vi "Teleop.vi"(10 "Match Info":T1={"Autonomous Elapsed Seconds"=0.0, "TeleOp Elapsed Seconds"=0.0, "Disabled Elapsed Seconds"=0.0, "Visited Autonomous"=FALSE, "Visited TeleOp"=FALSE, "Visited Disabled"=FALSE, "Autonomous Settings"={"Autonomous Style"=enum."Independent", "VI Refnum"=refnum}}, 11 "Call Context":T2) -> ()   [LabVIEW 2011]
doc: "This VI is called for each TeleOp packet received from the DS where the robot is not disabled. It is often used to read from the joysticks and update I/O or to update setpoints for timed control loops. It should complete and return within 20 milliseconds or it may miss DS packets."
uses:
  <vilib>/Rock Robotics/WPI/DriverStation/WPI_DriverStationDerivedRobotMode.ctl
  <vilib>/Rock Robotics/WPI/DriverStation/WPI_DriverStationMatch Info.ctl
  Robot Global Data.vi
panel:
  in  "Turret":dbl(knob)=0.008480890251286732 scale=-1.0..1.0
  out "Turret Output":dbl
  in  "Conveyor":dbl(knob) scale=-0.1..1.0
  out "Conveyor Output":dbl
  in  "Harvester":dbl(knob) scale=-1.0..1.0
  out "Harvester Output":dbl
  out "Shooter Output":dbl
  in  "Shooter":dbl(knob) scale=0.0..1.0
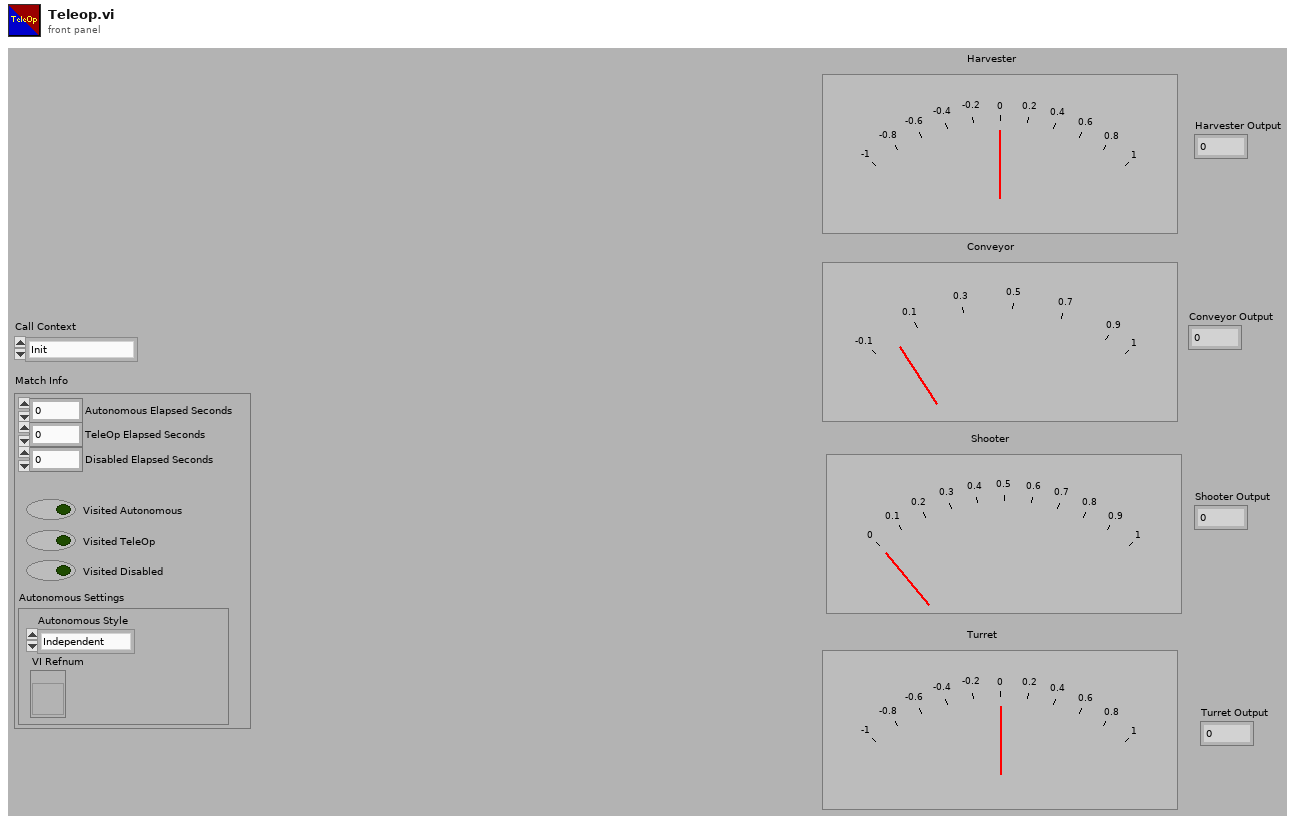
[diagram p1: front panel]
types:
  T1 = typedef "WPI_DriverStationMatch Info.ctl" = cluster{"Autonomous Elapsed Seconds":dbl, "TeleOp Elapsed Seconds":dbl, "Disabled Elapsed Seconds":dbl, "Visited Autonomous":bool, "Visited TeleOp":bool, "Visited Disabled":bool, "Autonomous Settings":cluster{"Autonomous Style":enum16{"Iterative", "Independent"}, "VI Refnum":refnum<vi>}}
  T2 = typedef "WPI_DriverStationDerivedRobotMode.ctl" = enum16{"Init", "Execute", "Stop"}
  T3 = typedef "WPI_JoystickDevRef.ctl" = cluster{"Device":T4}
  T4 = typedef "WPI_JoystickDeviceEnum.ctl" = enum16{"USB 1", "USB 2", "USB 3", "USB 4", "Kinect 1", "Kinect 2"}
  T5 = typedef "WPI_JoystickButtonState.ctl" = cluster{"Button 1":bool, "Button 2":bool, "Button 3":bool, "Button 4":bool, "Button 5":bool, "Button 6":bool, "Button 7":bool, "Button 8":bool, "Button 9":bool, "Button 10":bool, "Button 11":bool, "Button 12":bool}
  T6 = typedef "WPI_DigitalInputDevRef.ctl" = cluster{"DevStatus":errorcluster, "DIO Channel":T7, "Digital Module":T8}
  T7 = typedef "FPGA_DIOChannel.ctl" = enum8{"DIO 1", "DIO 2", "DIO 3", "DIO 4", "DIO 5", "DIO 6", "DIO 7", "DIO 8", "DIO 9", "DIO 10", "DIO 11", "DIO 12", "DIO 13", "DIO 14", "Invalid"}
  T8 = typedef "FPGA_TypedefDigitalModule.ctl" = enum16{"Digital Module 1", "Digital Module 2"}
  T9 = cluster{"Driver Station Digital Output (1-8)[0]":bool, "Driver Station Digital Output (1-8)[1]":bool, "Driver Station Digital Output (1-8)[2]":bool, "Driver Station Digital Output (1-8)[3]":bool, "Driver Station Digital Output (1-8)[4]":bool, "Driver Station Digital Output (1-8)[5]":bool, "Driver Station Digital Output (1-8)[6]":bool, "Driver Station Digital Output (1-8)[7]":bool, "Driver Station Digital Output (1-8)[8]":bool}
  T10 = cluster{"axis 1 (x)":dbl, "axis 2 (y)":dbl, "axis 3 (throttle)":dbl, "axis 4":dbl, "axis 5":dbl, "axis 6":dbl}
  T11 = typedef "WPI_ServoDeviceRef.ctl" = cluster{"DeviceStatus":errorcluster, "Digital Module":T8, "PWM Channel":T12, "DeadBand":T13}
  T12 = typedef "FPGA_DIOPWMChannel.ctl" = enum8{"PWM 1", "PWM 2", "PWM 3", "PWM 4", "PWM 5", "PWM 6", "PWM 7", "PWM 8", "PWM 9", "PWM 10", "Invalid"}
  T13 = typedef "WPI_PWMDeadband.ctl" = cluster{"Name":string, "maxPositivePwm":i32, "minPositivePwm":i32, "centerPwm":i32, "maxNegativePwm":i32, "minNegativePwm":i32, "angularRange":u16}
  T14 = typedef "WPI_MotorControlDeviceRef.ctl" = cluster{"DeviceStatus":errorcluster, "Type":enum16{"PWM", "CAN"}, "PWM":cluster{"Digital Module":T8, "PWM Channel":T12, "DeadBand":T13}, "CAN":cluster{"Device Number":u8, "Control Mode":T15, "Semaphore":T16, "Max Vout":dbl}, "Invert":bool, "TransformRef":T17, "InvTransformRef":T17}
  T15 = typedef "WPI_CANJaguar_ControlMode.ctl" = enum8{"Percent VBus", "Current", "Speed", "Position", "Voltage"}
  T16 = typedef "Semaphore RefNum" = refnum<k1>
  T17 = typedef "WPI_PWMTransform_ConPane.ctl" = refnum<vi>
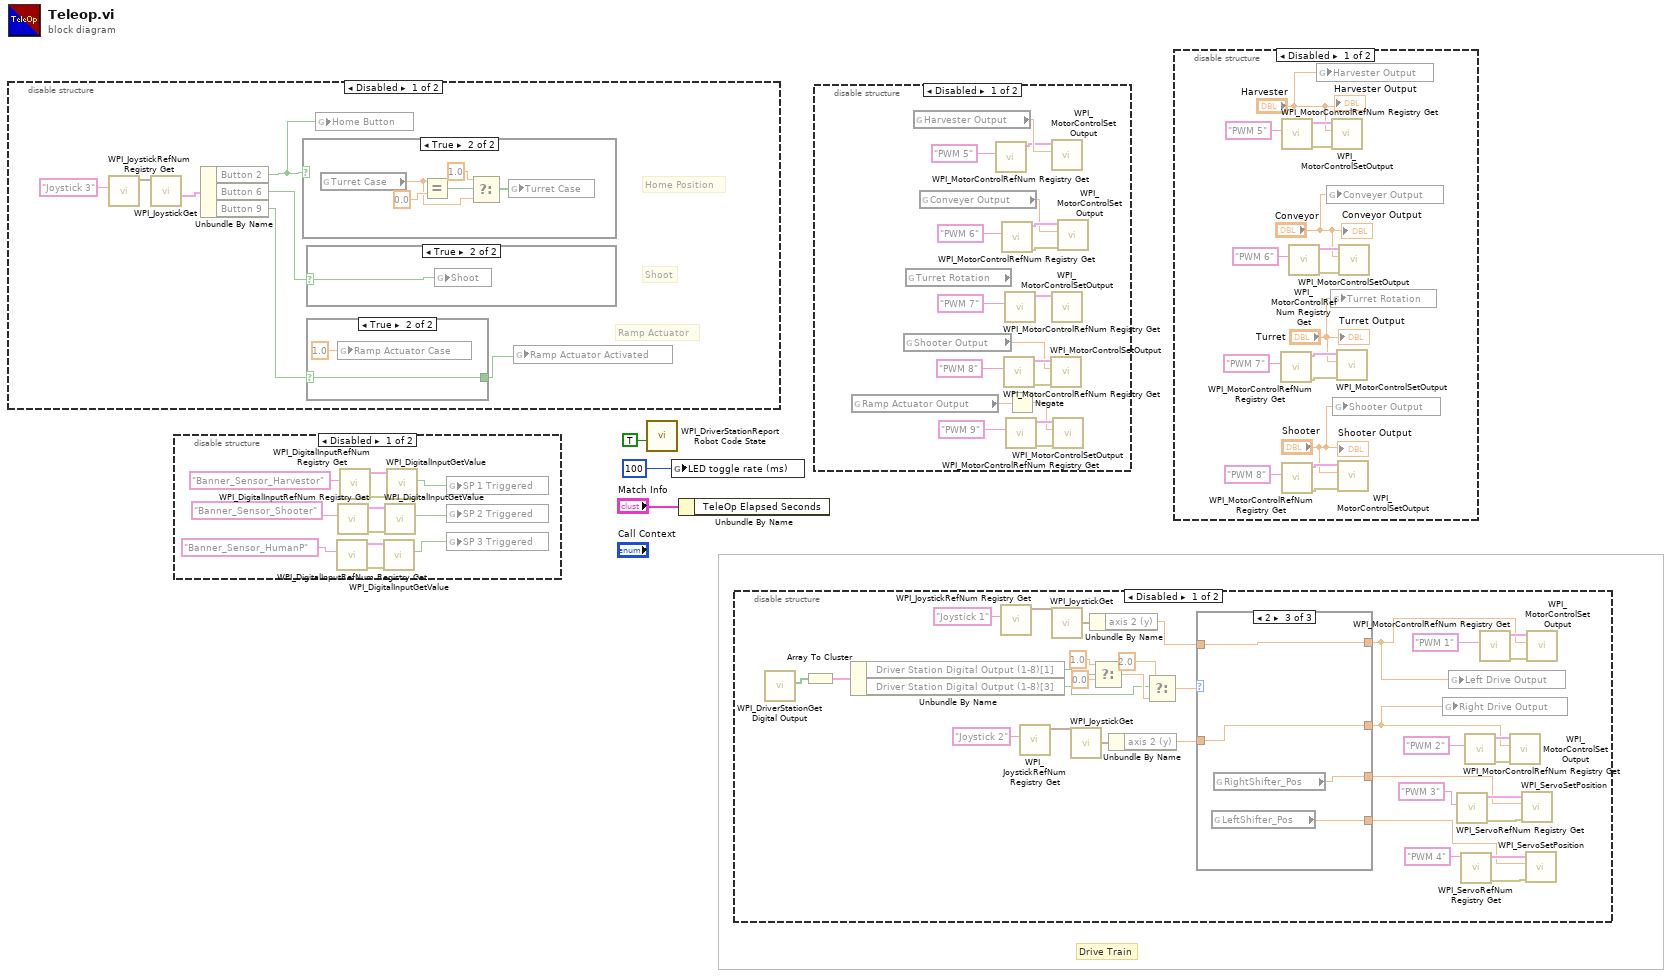
[diagram p0: block diagram]
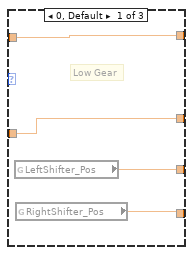
[diagram p3: hidden frame]
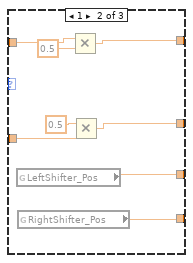
[diagram p4: hidden frame]
diagram:
  # "Drive Train"
  n1 = disable-structure shown="Disabled" {
    frame Disabled {
      # "Ramp Actuator"
      # "Shoot"
      # "Home Position"
      n2 = call <vilib>:"WPI_JoystickRefNum Registry Get.vi"("refnum name"="Joystick 3") -> ("JoystickDevRef"=w7:T3)  [unwired: 9 in, 1 out]
      n3 = call <vilib>:"WPI_JoystickGet.vi"("JoystickDevRef"=w7) -> ("Buttons"=w8:T5)  [unwired: 4 in, 2 out]
      n4 = Unbundle By Name(w8) -> ("Button 2"=w6:bool, "Button 6"=w5:bool, "Button 9"=w4:bool)
      n5 = case shown="True" w6 {
        frame False {
        }
        frame True {
          n6 = global read "Robot Global Data.vi" "Turret Case"() -> (w12:dbl)
          n7 = Equal?(x=w12, y=0.0) -> (x = y?=w14:bool)
          n8 = Select(t=1.0, s=w14, f=w12) -> (s? t:f=w11:dbl)
          n9 = global write "Robot Global Data.vi" "Turret Case"(w11) -> ()
        }
      }
      n10 = case shown="True" w5 {
        selector: w5 -> [_ w16]
        frame False {
        }
        frame True {
          n11 = global write "Robot Global Data.vi" "Shoot"(w16) -> ()
        }
      }
      n12 = case shown="True" w4 {
        selector: w4 -> [w17 w19]
        tunnel: [w17 w19] -> w10
        frame False {
        }
        frame True {
          n13 = global write "Robot Global Data.vi" "Ramp Actuator Case"(1.0 ("Ramp Actuator Case")) -> ()
        }
      }
      n14 = global write "Robot Global Data.vi" "Home Button"(w6) -> ()
      n15 = global write "Robot Global Data.vi" "Ramp Actuator Activated"(w10) -> ()
    }
    frame Enabled {
    }
  }
  n16 = disable-structure shown="Disabled" {
    frame Disabled {
      n17 = call <vilib>:"WPI_DigitalInputRefNum Registry Get.vi"("refnum name"="Banner_Sensor_HumanP") -> ("error out"=w26:errorcluster, "DigitalInputDevRef"=w25:T6)  [unwired: 9 in]
      n18 = call <vilib>:"WPI_DigitalInputRefNum Registry Get.vi"("refnum name"="Banner_Sensor_Shooter") -> ("error out"=w27:errorcluster, "DigitalInputDevRef"=w28:T6)  [unwired: 9 in]
      n19 = call <vilib>:"WPI_DigitalInputRefNum Registry Get.vi"("refnum name"="Banner_Sensor_Harvestor") -> ("error out"=w31:errorcluster, "DigitalInputDevRef"=w30:T6)  [unwired: 9 in]
      n20 = call <vilib>:"WPI_DigitalInputGetValue.vi"("error in (no error)"=w26, "DigitalInputDevRef"=w25) -> ("Value"=w23:bool)  [unwired: 7 in, 2 out]
      n21 = call <vilib>:"WPI_DigitalInputGetValue.vi"("error in (no error)"=w27, "DigitalInputDevRef"=w28) -> ("Value"=w24:bool)  [unwired: 7 in, 2 out]
      n22 = call <vilib>:"WPI_DigitalInputGetValue.vi"("error in (no error)"=w31, "DigitalInputDevRef"=w30) -> ("Value"=w29:bool)  [unwired: 7 in, 2 out]
      n23 = global write "Robot Global Data.vi" "SP 1 Triggered"(w29) -> ()
      n24 = global write "Robot Global Data.vi" "SP 2 Triggered"(w24) -> ()
      n25 = global write "Robot Global Data.vi" "SP 3 Triggered"(w23) -> ()
    }
    frame Enabled {
    }
  }
  n26 = call <vilib>:"WPI_DriverStationReport Robot Code State.vi"("TeleOp"=TRUE ("Autonomous")) -> ()  [unwired: 10 in, 1 out]
  n27 = global write "Robot Global Data.vi" "LED toggle rate (ms)"(u32 100 ("LED ms toggle rate")) -> ()
  n28 = Unbundle By Name("Match Info") -> ()  [unwired: 1 out]
  n29 = disable-structure shown="Disabled" {
    frame Disabled {
      n30 = call <vilib>:"WPI_DriverStationGet Digital Output.vi"() -> ("Driver Station Digital Output (1-8)"=w64:bool[])  [unwired: 10 in, 1 out]
      n31 = Array To Cluster(array=w64) -> (cluster=w63:T9)
      n32 = Unbundle By Name(w63) -> ("Driver Station Digital Output (1-8)[1]"=w32:bool, "Driver Station Digital Output (1-8)[3]"=w59:bool)
      n33 = call <vilib>:"WPI_JoystickRefNum Registry Get.vi"("refnum name"="Joystick 1") -> ("JoystickDevRef"=w55:T3)  [unwired: 9 in, 1 out]
      n34 = call <vilib>:"WPI_JoystickRefNum Registry Get.vi"("refnum name"="Joystick 2") -> ("JoystickDevRef"=w52:T3)  [unwired: 9 in, 1 out]
      n35 = call <vilib>:"WPI_JoystickGet.vi"("JoystickDevRef"=w55) -> ("Axes"=w54:T10)  [unwired: 4 in, 2 out]
      n36 = call <vilib>:"WPI_JoystickGet.vi"("JoystickDevRef"=w52) -> ("Axes"=w53:T10)  [unwired: 4 in, 2 out]
      n37 = Unbundle By Name(w54) -> ("axis 2 (y)"=w49:dbl)
      n38 = Select(t=1.0, s=w32, f=0.0 ("t")) -> (s? t:f=w60:dbl)
      n39 = Unbundle By Name(w53) -> ("axis 2 (y)"=w50:dbl)
      n40 = Select(t=2.0, s=w59, f=w60) -> (s? t:f=w57:dbl)
      n41 = case shown="2" w57 {
        tunnel: w50 -> [w68 w72 w79]
        tunnel: w49 -> [w67 w75 w80]
        tunnel: [w68 w73 w79] -> w41
        tunnel: [w67 w74 w80] -> w42
        tunnel: [w66 w69 w78] -> w34
        tunnel: [w65 w70 w77] -> w33
        frame 0, Default {
          # "Low Gear"
          n42 = global read "Robot Global Data.vi" "LeftShifter_Pos"() -> (w66:dbl)
          n43 = global read "Robot Global Data.vi" "RightShifter_Pos"() -> (w65:dbl)
        }
        frame 1 {
          n44 = global read "Robot Global Data.vi" "LeftShifter_Pos"() -> (w69:dbl)
          n45 = global read "Robot Global Data.vi" "RightShifter_Pos"() -> (w70:dbl)
          n46 = Multiply(x=w75, y=0.5) -> (x*y=w74:dbl)
          n47 = Multiply(x=0.5 ("y"), y=w72) -> (x*y=w73:dbl)
        }
        frame 2 {
          n48 = global read "Robot Global Data.vi" "LeftShifter_Pos"() -> (w77:dbl)
          n49 = global read "Robot Global Data.vi" "RightShifter_Pos"() -> (w78:dbl)
        }
      }
      n50 = global write "Robot Global Data.vi" "Right Drive Output"(w41) -> ()
      n51 = global write "Robot Global Data.vi" "Left Drive Output"(w42) -> ()
      n52 = call <vilib>:"WPI_ServoRefNum Registry Get.vi"("refnum name"="PWM 3") -> ("error out"=w38:errorcluster, "ServoDeviceRef"=w39:T11)  [unwired: 9 in]
      n53 = call <vilib>:"WPI_ServoRefNum Registry Get.vi"("refnum name"="PWM 4") -> ("error out"=w37:errorcluster, "ServoDeviceRef"=w36:T11)  [unwired: 9 in]
      n54 = call <vilib>:"WPI_MotorControlRefNum Registry Get.vi"("refnum name"="PWM 2") -> ("error out"=w43:errorcluster, "MotorControlDevRef"=w44:T14)  [unwired: 9 in]
      n55 = call <vilib>:"WPI_MotorControlRefNum Registry Get.vi"("refnum name"="PWM 1") -> ("error out"=w45:errorcluster, "MotorControlDevRef"=w46:T14)  [unwired: 9 in]
      n56 = call <vilib>:"WPI_MotorControlSetOutput.vi"("error in (no error)"=w43, "Output"=w41, "MotorControlDevRef"=w44) -> ()  [unwired: 7 in, 2 out]
      n57 = call <vilib>:"WPI_ServoSetPosition.vi"("error in (no error)"=w38, "Position"=w34, "ServoDeviceRef"=w39) -> ()  [unwired: 7 in, 2 out]
      n58 = call <vilib>:"WPI_ServoSetPosition.vi"("error in (no error)"=w37, "Position"=w33, "ServoDeviceRef"=w36) -> ()  [unwired: 7 in, 2 out]
      n59 = call <vilib>:"WPI_MotorControlSetOutput.vi"("error in (no error)"=w45, "Output"=w42, "MotorControlDevRef"=w46) -> ()  [unwired: 7 in, 2 out]
    }
    frame Enabled {
    }
  }
  n60 = disable-structure shown="Disabled" {
    frame Disabled {
      n61 = global read "Robot Global Data.vi" "Ramp Actuator Output"() -> (w94:dbl)
      n62 = global read "Robot Global Data.vi" "Shooter Output"() -> (w86:dbl)
      n63 = global read "Robot Global Data.vi" "Turret Rotation"() -> ()  [unwired: 1 out]
      n64 = global read "Robot Global Data.vi" "Harvester Output"() -> (w83:dbl)
      n65 = global read "Robot Global Data.vi" "Conveyer Output"() -> (w90:dbl)
      n66 = call <vilib>:"WPI_MotorControlRefNum Registry Get.vi"("refnum name"="PWM 5") -> ("MotorControlDevRef"=w81:T14)  [unwired: 9 in, 1 out]
      n67 = call <vilib>:"WPI_MotorControlRefNum Registry Get.vi"("refnum name"="PWM 6") -> ("error out"=w93:errorcluster, "MotorControlDevRef"=w92:T14)  [unwired: 9 in]
      n68 = call <vilib>:"WPI_MotorControlRefNum Registry Get.vi"("refnum name"="PWM 8") -> ("error out"=w88:errorcluster, "MotorControlDevRef"=w89:T14)  [unwired: 9 in]
      n69 = call <vilib>:"WPI_MotorControlRefNum Registry Get.vi"("refnum name"="PWM 7") -> ("MotorControlDevRef"=w85:T14)  [unwired: 9 in, 1 out]
      n70 = call <vilib>:"WPI_MotorControlRefNum Registry Get.vi"("refnum name"="PWM 9") -> ("error out"=w97:errorcluster, "MotorControlDevRef"=w96:T14)  [unwired: 9 in]
      n71 = Negate(x=w94) -> (-x=w95:dbl)
      n72 = call <vilib>:"WPI_MotorControlSetOutput.vi"("error in (no error)"=w88, "Output"=w86, "MotorControlDevRef"=w89) -> ()  [unwired: 7 in, 2 out]
      n73 = call <vilib>:"WPI_MotorControlSetOutput.vi"("Output"=w83, "MotorControlDevRef"=w81) -> ()  [unwired: 8 in, 2 out]
      n74 = call <vilib>:"WPI_MotorControlSetOutput.vi"("MotorControlDevRef"=w85) -> ()  [unwired: 9 in, 2 out]
      n75 = call <vilib>:"WPI_MotorControlSetOutput.vi"("error in (no error)"=w97, "Output"=w95, "MotorControlDevRef"=w96) -> ()  [unwired: 7 in, 2 out]
      n76 = call <vilib>:"WPI_MotorControlSetOutput.vi"("error in (no error)"=w93, "Output"=w90, "MotorControlDevRef"=w92) -> ()  [unwired: 7 in, 2 out]
    }
    frame Enabled {
    }
  }
  n77 = disable-structure shown="Disabled" {
    frame Disabled {
      n78 = call <vilib>:"WPI_MotorControlRefNum Registry Get.vi"("refnum name"="PWM 7") -> ("error out"=w105:errorcluster, "MotorControlDevRef"=w104:T14)  [unwired: 9 in]
      n79 = call <vilib>:"WPI_MotorControlRefNum Registry Get.vi"("refnum name"="PWM 5") -> ("error out"=w107:errorcluster, "MotorControlDevRef"=w108:T14)  [unwired: 9 in]
      n80 = call <vilib>:"WPI_MotorControlRefNum Registry Get.vi"("refnum name"="PWM 8") -> ("error out"=w112:errorcluster, "MotorControlDevRef"=w113:T14)  [unwired: 9 in]
      n81 = call <vilib>:"WPI_MotorControlRefNum Registry Get.vi"("refnum name"="PWM 6") -> ("error out"=w110:errorcluster, "MotorControlDevRef"=w111:T14)  [unwired: 9 in]
      n82 = global write "Robot Global Data.vi" "Harvester Output"("Harvester") -> ()
      n83 = global write "Robot Global Data.vi" "Conveyer Output"("Conveyor") -> ()
      n84 = global write "Robot Global Data.vi" "Turret Rotation"("Turret") -> ()
      n85 = call <vilib>:"WPI_MotorControlSetOutput.vi"("error in (no error)"=w107, "Output"="Harvester", "MotorControlDevRef"=w108) -> ()  [unwired: 7 in, 2 out]
      n86 = global write "Robot Global Data.vi" "Shooter Output"("Shooter") -> ()
      n87 = call <vilib>:"WPI_MotorControlSetOutput.vi"("error in (no error)"=w105, "Output"="Turret", "MotorControlDevRef"=w104) -> ()  [unwired: 7 in, 2 out]
      n88 = call <vilib>:"WPI_MotorControlSetOutput.vi"("error in (no error)"=w112, "Output"="Shooter", "MotorControlDevRef"=w113) -> ()  [unwired: 7 in, 2 out]
      n89 = call <vilib>:"WPI_MotorControlSetOutput.vi"("error in (no error)"=w110, "Output"="Conveyor", "MotorControlDevRef"=w111) -> ()  [unwired: 7 in, 2 out]
      "Shooter Output" <- "Shooter"
      "Harvester Output" <- "Harvester"
      "Conveyor Output" <- "Conveyor"
      "Turret Output" <- "Turret"
    }
    frame Enabled {
    }
  }
